vi "AprilTagFieldLayout_GetTagPose.vi"(9 "TagId":i32, 11 "AprilTagFieldLayout":T5={"AprilTagMap"={}, "FieldLength"=0.0, "FieldWidth"=0.0, "OriginPosition "=enum."kBlueAllianceWallRightSide,", "OriginPose3d"={"Translation3d"={"X"=0.0, "Y"=0.0, "Z"=0.0}, "Rotation3d"={"Q_quaternion"={"R"=1.0, "V"=[0.0, 0.0, 0.0]}}}} {"OriginPose3d"."Translation3d"."Z" format="%14.3f"; "OriginPose3d"."Translation3d"."Y" format="%14.3f"; "OriginPose3d"."Translation3d"."X" format="%14.3f"}) -> (1 "Found":bool, 3 "TagPose3d":T1={"Translation3d"={"X"=0.0, "Y"=0.0, "Z"=0.0}, "Rotation3d"={"Q_quaternion"={"R"=1.0, "V"=[0.0, 0.0, 0.0]}}} {"Translation3d"."Z" format="%14.3f"; "Translation3d"."Y" format="%14.3f"; "Translation3d"."X" format="%14.3f"})   [LabVIEW 2019, in "Trajectory_Library.lvlib"]
doc: "Returns the location of a particular AprilTag on the field. \n\nInputs:\n -- AprilTagFIeldLayout -- AprilTagFieldLayout -- Data cluster \n -- TagID -- Integer -- The AprilTag to locate.\n\nOutputs:\n -- TagPose3d -- Pose3d -- Location of the AprilTag. This is relative to the specifc origin specified in the AprilTagFieldLayout. \n -- Found -- Boolean -- TRUE if the TagID was found in the field definition."
uses:
  Trajectory_Library.lvlib
  TypeDef/AprilTagFieldLayout.ctl
  TypeDef/AprilTag.ctl
  TypeDef/POSE3D.ctl
  TypeDef/TRANSLATION3D.ctl
  TypeDef/ROTATION3D.ctl
  TypeDef/QUATERNION.ctl
  Enum/AprilTagFieldLayoutOrignPosition_ENUM.ctl
  Pose3d_New_Trans3dRot3d.vi
  Transform3d_Create_Pose3dPose3d.vi
  Transform3d_GetRotation3d.vi
  Transform3d_GetTranslation3d.vi
  Transform3d_Create_Trans3dRot3d.vi
  Translation3d_Minus.vi
  Translation3d_RotateBy.vi
  Rotation3d_UnaryMinus.vi
  Pose3d_getTranslation3d.vi
  Pose3d_getRotation3d.vi
  Rotation3d_Minus.vi
  Translation3d_Create.vi
  Rotation3d_GetQuaterion.vi
  Quaternion_New.vi
  Quaternion_Times.vi
  Quaternion_Inverse.vi
  Quaternion_Get_All.vi
  Rotation3d_Create_Quaternion.vi
  Rotation3d_RotateBy.vi
  Quaternion_Normalize.vi
  Quaternion_New_Default.vi
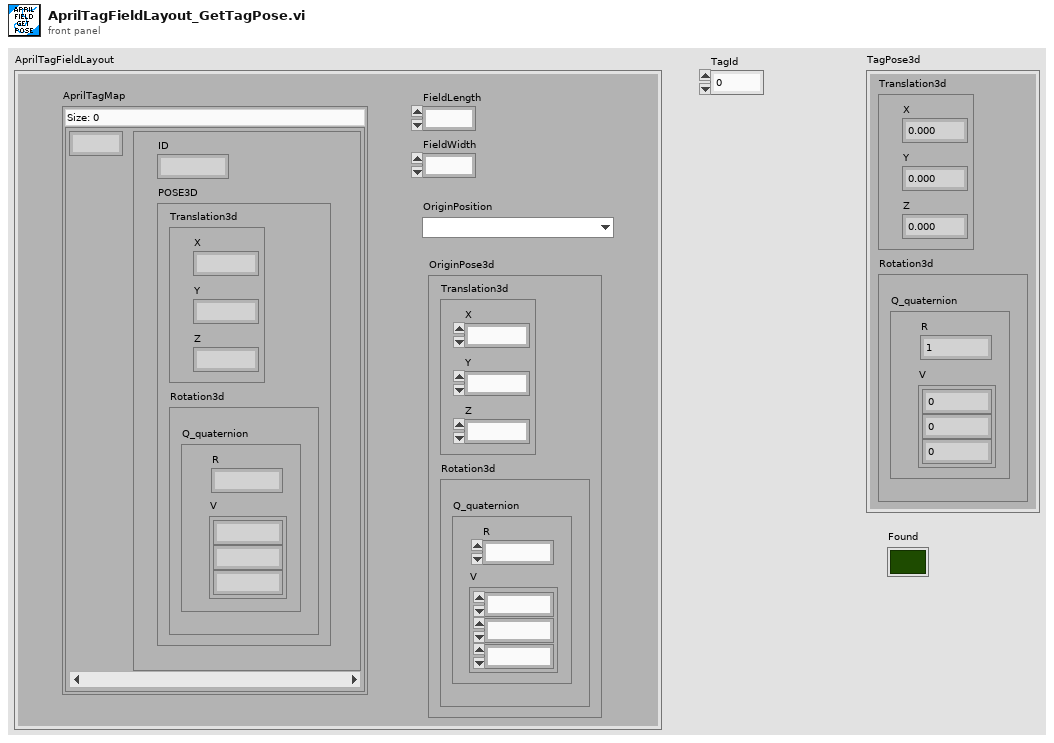
[diagram p1: front panel]
types:
  T1 = typedef "Trajectory_Library.lvlib/POSE3D.ctl" = cluster{"Translation3d":T2, "Rotation3d":T3}
  T2 = typedef "Trajectory_Library.lvlib/TRANSLATION3D.ctl" = cluster{"X":dbl, "Y":dbl, "Z":dbl}
  T3 = typedef "Trajectory_Library.lvlib/ROTATION3D.ctl" = cluster{"Q_quaternion":T4}
  T4 = typedef "Trajectory_Library.lvlib/QUATERNION.ctl" = cluster{"R":dbl, "V":dbl[]}
  T5 = typedef "Trajectory_Library.lvlib/AprilTagFieldLayout.ctl" = cluster{"AprilTagMap":map{i32, T6}, "FieldLength":dbl, "FieldWidth":dbl, "OriginPosition ":T7, "OriginPose3d":T1}
  T6 = typedef "Trajectory_Library.lvlib/AprilTag.ctl" = cluster{"ID":i32, "POSE3D":T1}
  T7 = typedef "Trajectory_Library.lvlib/AprilTagFieldLayoutOrignPosition_ENUM.ctl" = enum16{"kBlueAllianceWallRightSide,", "kRedAllianceWallRightSide,"}
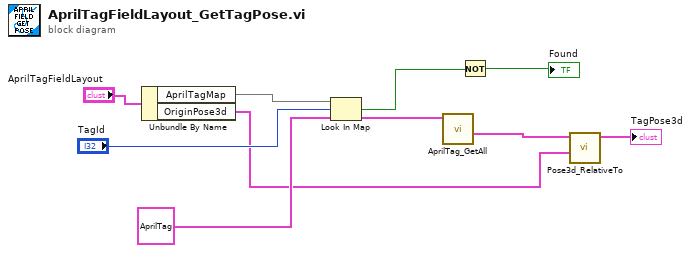
[diagram p0: block diagram]
diagram:
  n1 = Unbundle By Name("AprilTagFieldLayout") -> ("AprilTagMap"=w9:map{i32, T6}, "OriginPose3d"=w2:T1)
  n2 = Look In Map(map=w9, key="TagId", default value=T6 {"ID"=0, "POSE3D"={"Translation3d"={"X"=0.0, "Y"=0.0, "Z"=0.0}, "Rotation3d"={"Q_quaternion"={"R"=1.0, "V"=[0.0, 0.0, 0.0]}}}}) -> (key not found?=w6:bool, value=w4:T6)
  n3 = call "AprilTag_GetAll.vi"("AprilTag"=w4) -> ("POSE3D"=w3:T1)  [unwired: 9 in, 1 out]
  n4 = Not(x=w6) -> (.not. x?=→"Found":bool)
  n5 = call "Pose3d_RelativeTo.vi"("other Pose3d"=w2, "in Pose3d"=w3) -> ("out Pose3d"=→"TagPose3d":T1)  [unwired: 9 in]
